vi "Get Execution Paused.vi"(8 "error in (no error)":errorcluster, 11 "Status Monitor in":T1) -> (0 "error out":errorcluster, 3 "Paused?":bool)   [LabVIEW 2023, in "HardwareAbstractionLayer_LVOOP.lvlib" / "Teststand.lvclass"]
uses:
  Teststand.lvclass
  <vilib>/addons/TestStand/_TSUtility.llb/TestStand - Status Monitor.ctl
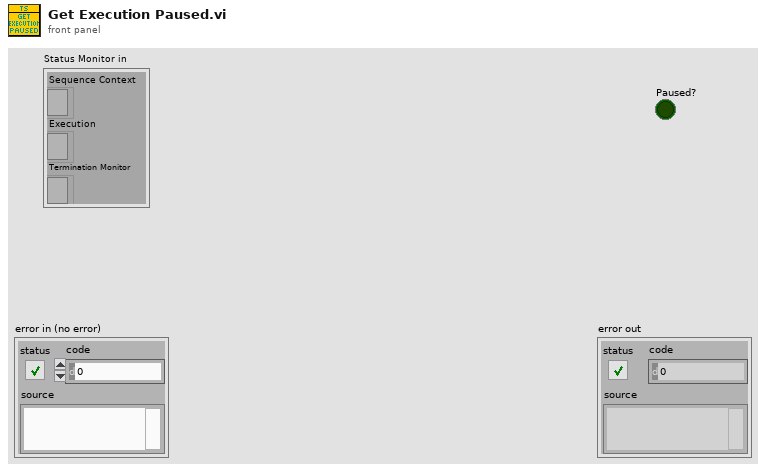
[diagram p1: front panel]
types:
  T1 = typedef "TestStand - Status Monitor.ctl" = cluster{"Sequence Context":refnum<k7>, "Execution":refnum<k7>, "Termination Monitor":refnum<k7>}
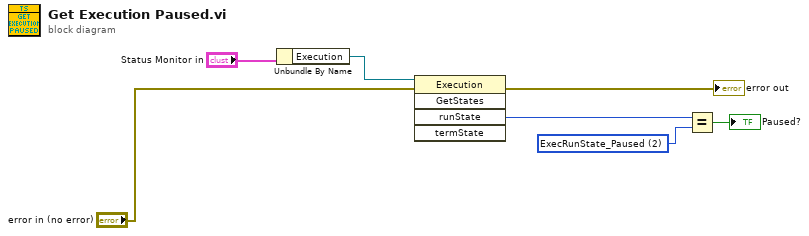
[diagram p0: block diagram]
diagram:
  w6 = 2 items=["ExecRunState_Running"=1, "ExecRunState_Paused"=2, "ExecRunState_Stopped"=3] ("runState")
  n1 = Unbundle By Name("Status Monitor in") -> ("Execution"=w1:refnum<k7>)
  n2 = invoke class="Execution" method="GetStates"(reference=w1, error in="error in (no error)") -> (error out=→"error out":errorcluster, "runState"=w7:i32)  [unwired: 3 in, 3 out]
  n3 = Equal?(x=w7, y=w6) -> (x = y?=→"Paused?":bool)
